vi "read current amp.vi"(8 "error in":errorcluster, 11 "Coarse Approach in":refnum<class "Coarse Approach.lvclass">) -> (0 "error out":errorcluster, 1 "Z Voltage out":i16(slide) scale=32767.0..-32768.0, 2 "Amplitude (V rms)":dbl, 3 "Coarse Approach out":refnum<class "Coarse Approach.lvclass">)   [LabVIEW 2020, in "Coarse Approach.lvclass"]
uses:
  Coarse Approach.lvclass
  Coarse Approach.lvclass/Coarse Approach.ctl
  Lock-In Amplifier/Lock-In Amplifier.lvclass
  PZT/PZT.lvclass
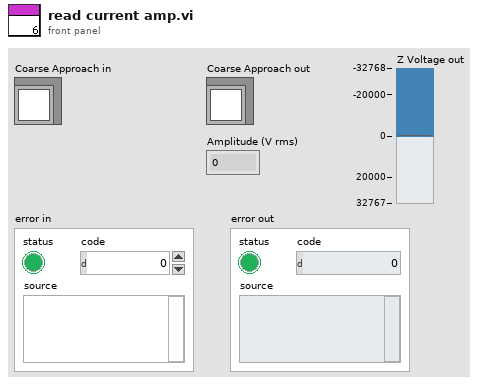
[diagram p1: front panel]
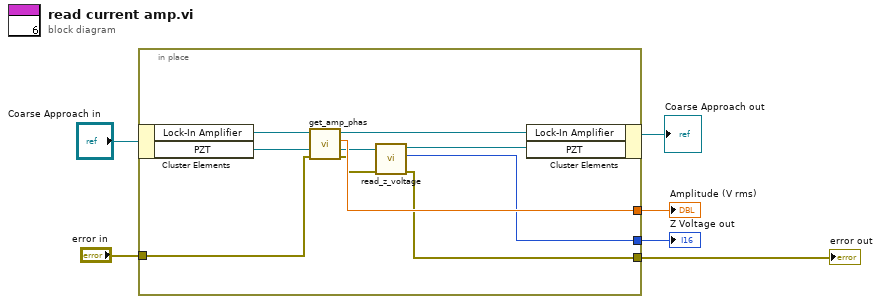
[diagram p0: block diagram]
diagram:
  n1 = in-place {
    in-place-border: [w13] -> w4
    in-place-border: "error in" -> [w10]
    in-place-border: [w8] -> w1
    in-place-border: [w7] -> w2
    n2 = in-place-cluster #1("Coarse Approach in") -> ("Lock-In Amplifier"=w15:refnum<class "Lock-In Amplifier.lvclass">, "PZT"=w12:refnum<class "PZT.lvclass">)
    n3 = call-dynamic "get_amp_phas.vi"("error in (no error)"=w10, "Lock-In Amplifier in"=w15) -> ("error out"=w9:errorcluster, "Amplitude (V rms)"=w13:dbl, "Lock-In Amplifier out"=w14:refnum<class "Lock-In Amplifier.lvclass">)  [unwired: 6 in, 1 out]
    n4 = call "read_z_voltage.vi"("error in"=w9, "PZT in"=w12) -> ("error out"=w8:errorcluster, "Z Voltage out"=w7:i16, "PZT out"=w11:refnum<class "PZT.lvclass">)  [unwired: 7 in]
    n5 = in-place-cluster #1("Lock-In Amplifier"=w14, "PZT"=w11) -> (→"Coarse Approach out":refnum<class "Coarse Approach.lvclass">)
  }
  "Amplitude (V rms)" <- w4
  "error out" <- w1
  "Z Voltage out" <- w2
